vi "Combine message parts.vi"(7 "Data":u8[](array[numeric]), 9 "part":u8, 12 "Expected bytes":i32) -> (8 "Data complete":u8[](array[numeric]), 10 "Complete data":bool)   [LabVIEW 2011]
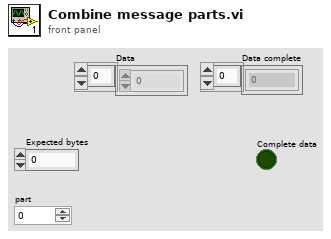
[diagram p1: front panel]
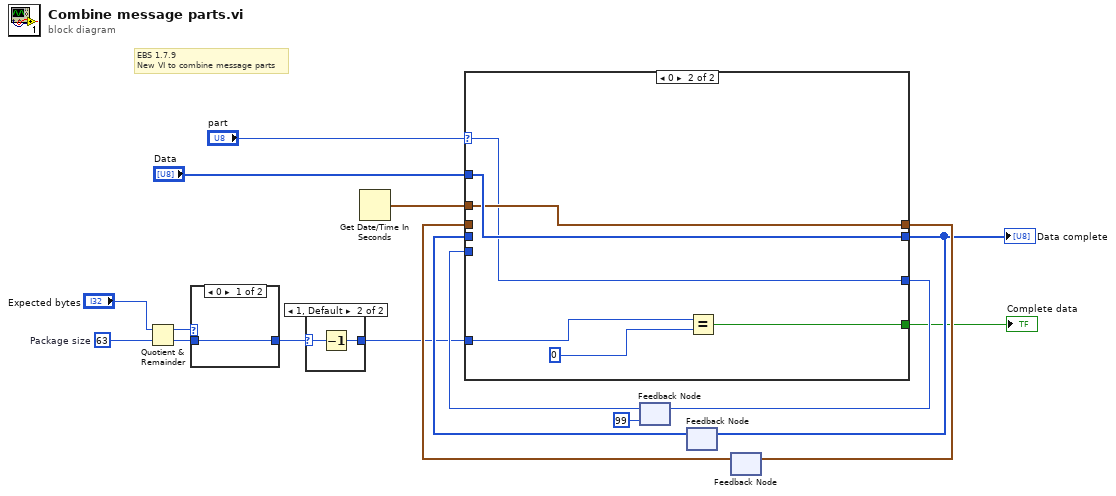
[diagram p0: block diagram]
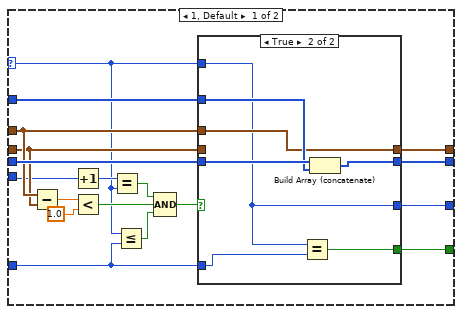
[diagram p3: hidden frame]
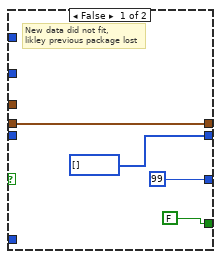
[diagram p4: hidden frame]
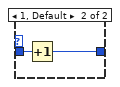
[diagram p5: hidden frame]
diagram:
  w2 = 63  # Package size
  # "EBS 1.7.9 \nNew VI to combine message parts"
  n1 = Quotient & Remainder(x="Expected bytes", y=w2) -> (x-y*floor(x/y)=w9:i32, floor(x/y)=w10:i32)
  n2 = case shown="0" w9 {
    tunnel: w10 -> [w18 w20]
    tunnel: [w18 w19] -> w1
    frame 0 {
    }
    frame 1, Default {
      n3 = Increment(x=w20) -> (x+1=w19:i32)
    }
  }
  n4 = case shown="1, Default" w1 {
    selector: w1 -> [w21 w22]
    tunnel: [w21 w23] -> w4
    frame 0 {
    }
    frame 1, Default {
      n5 = Decrement(x=w22) -> (x-1=w23:i32)
    }
  }
  n6 = Get Date/Time In Seconds() -> (seconds since 1Jan1904=w16:timestamp)
  n7 = feedback #1(u8 99 ("part")) -> (w8:u8)
  n8 = feedback #2() -> (w13:u8[])  [unwired: 1 in]
  n9 = feedback #3() -> (w15:timestamp)  [unwired: 1 in]
  n10 = case shown="0" "part" {
    selector: "part" -> [w26 w56]
    tunnel: "Data" -> [w40 w58]
    tunnel: [w39 w58] -> w12
    tunnel: w13 -> [w41 _]
    tunnel: [w34 w57] -> w14
    tunnel: w15 -> [w35 _]
    tunnel: w16 -> [w36 w57]
    tunnel: [w33 w56] -> w17
    tunnel: w8 -> [w32 _]
    tunnel: w4 -> [w24 w55]
    tunnel: [w25 w53] -> w6
    frame 1, Default {
      n11 = Subtract(x=w36, y=w35) -> (x-y=w38:dbl)
      n12 = Increment(x=w32) -> (x+1=w31:u8)
      n13 = Less?(x=w38, y=1.0) -> (x < y?=w29:bool)
      n14 = Equal?(x=w31, y=w26) -> (x = y?=w30:bool)
      n15 = Less Or Equal?(x=w26, y=w24) -> (x <= y?=w28:bool)
      n16 = Compound Arithmetic op=AND(w30, w29, w28) -> (w27:bool)
      n17 = case shown="True" w27 {
        tunnel: w41 -> [_ w52]
        tunnel: w40 -> [_ w51]
        tunnel: [u8[] [] w50] -> w39
        tunnel: w36 -> [_ w49]
        tunnel: w35 -> [w43 _]
        tunnel: [w43 w49] -> w34
        tunnel: [u8 99 ("part") w48] -> w33
        tunnel: w26 -> [_ w48]
        tunnel: [FALSE w46] -> w25
        tunnel: w24 -> [_ w47]
        frame False {
          # "New data did not fit, \nlikley previous package lost"
        }
        frame True {
          n18 = Equal?(x=w48, y=w47) -> (x = y?=w46:bool)
          n19 = Build Array (concatenate)(w52, w51) -> (w50:u8[])
        }
      }
    }
    frame 0 {
      n20 = Equal?(x=w55, y=0) -> (x = y?=w53:bool)
    }
  }
  "Data complete" <- w12
  "Complete data" <- w6
  n21 = feedback-in #1(w17) -> ()
  n22 = feedback-in #2(w12) -> ()
  n23 = feedback-in #3(w14) -> ()
